vi "Read Serial Configuration.vi"(8 "error in (no error)":errorcluster, 11 "MelsecFxLinks in":refnum<class "MelsecFxLinks.lvclass">) -> (0 "error out":errorcluster, 2 "Serial Configuration":T1 {"parity" items=["None", "Odd", "Even", "Mark", "Space"]; "stopBits" items=["None", "One", "Two", "OnePointFive"]}, 3 "MelsecFxLinks out":refnum<class "MelsecFxLinks.lvclass">)   [LabVIEW 2020, in "MelsecFxLinks.lvclass"]
uses:
  MelsecFxLinks.lvclass
  MelsecFxLinks.lvclass/MelsecFxLinks.ctl
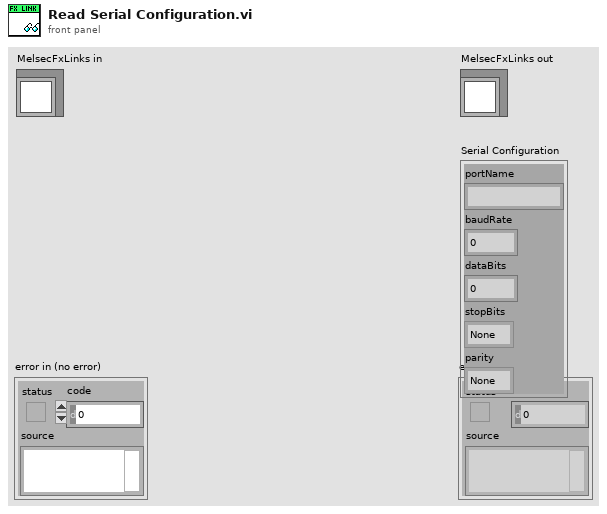
[diagram p1: front panel]
types:
  T1 = cluster{"portName":string, "baudRate":i32, "dataBits":i32, "stopBits":i32, "parity":i32}
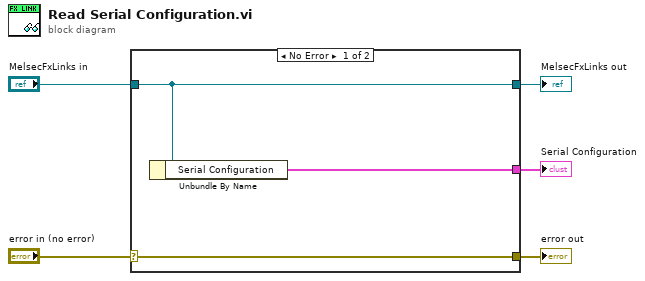
[diagram p0: block diagram]
diagram:
  n1 = case shown="No Error" "error in (no error)" {
    selector: "error in (no error)" -> [w8 w9]
    tunnel: [w8 w9] -> w4
    tunnel: [w7 w10] -> w2
    tunnel: "MelsecFxLinks in" -> [w7 w10]
    tunnel: [w6 _] -> w1
    frame No Error {
      n2 = Unbundle By Name(w7) -> ("Serial Configuration"=w6:T1)
    }
    frame Error {
    }
  }
  "error out" <- w4
  "MelsecFxLinks out" <- w2
  "Serial Configuration" <- w1
